vi "SetpointSetter.vi"() -> (1 "Arm Pos":T1, 3 "Shooter Servo Pos":T2)   [LabVIEW 2013]
uses:
  <vilib>/Utility/file.llb/Read From Spreadsheet File (DBL).vi
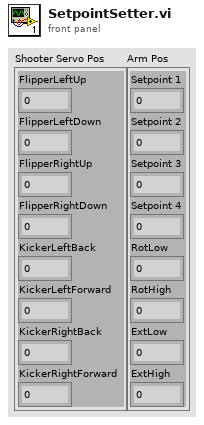
[diagram p1: front panel]
types:
  T1 = cluster{"Setpoint 1":dbl, "Setpoint 2":dbl, "Setpoint 3":dbl, "Setpoint 4":dbl, "RotLow":dbl, "RotHigh":dbl, "ExtLow":dbl, "ExtHigh":dbl}
  T2 = cluster{"FlipperLeftUp":dbl, "FlipperLeftDown":dbl, "FlipperRightUp":dbl, "FlipperRightDown":dbl, "KickerLeftBack":dbl, "KickerLeftForward":dbl, "KickerRightBack":dbl, "KickerRightForward":dbl}
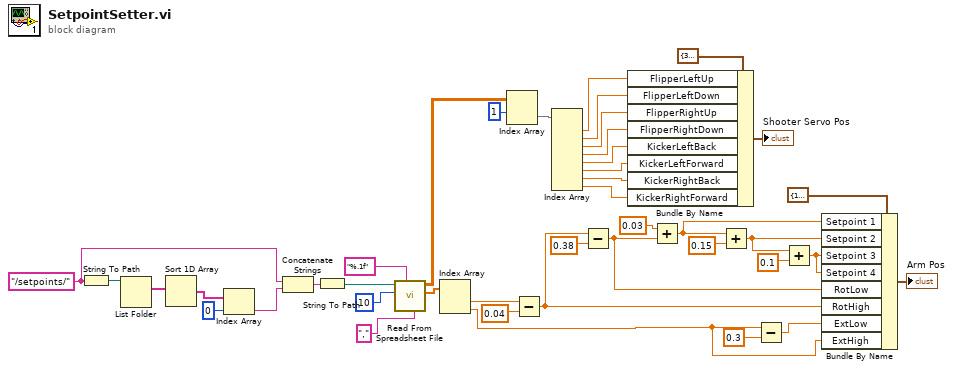
[diagram p0: block diagram]
diagram:
  w12 = "/setpoints/" ("string")
  n1 = String To Path(string=w12) -> (path=w10:path)
  n2 = List Folder(path=w10) -> (filenames=w9:string[])  [unwired: 1 in, 5 out]
  n3 = Sort 1D Array(array=w9) -> (sorted array=w8:string[])
  n4 = Index Array(array=w8, index=0) -> (element=w11:string)
  n5 = Concatenate Strings(w12, w11) -> (w6:string)
  n6 = String To Path(string=w6) -> (path=w7:path)
  n7 = call-poly <vilib>:"Read From Spreadsheet File.vi"("delimiter (\\t)"="," ("delimiter (\\t)"), "format (%.3f)"="%.1f", "number of rows (all:-1)"=10, "file path (dialog if empty)"=w7) -> ("first row"=w13:dbl[], "all rows"=w29:dbl[][])  [unwired: 1 in, 5 out]
  n8 = Index Array(array=w13) -> (element #1=w15:dbl, element #2=w28:dbl)  [unwired: 2 in]
  n9 = Index Array(array=w29, index (row)=1) -> (element=w32:dbl[])  [unwired: 1 in]
  n10 = Subtract(x=w15, y=0.04) -> (x-y=w17:dbl)
  n11 = Index Array(array=w32) -> (element #1=w33:dbl, element #2=w34:dbl, element #3=w35:dbl, element #4=w36:dbl, element #5=w37:dbl, element #6=w38:dbl, element #7=w39:dbl, element #8=w40:dbl)  [unwired: 8 in]
  n12 = Subtract(x=w17, y=0.38) -> (x-y=w19:dbl)
  n13 = Bundle By Name(cluster=T2 {"FlipperLeftUp"=30.0, "FlipperLeftDown"=115.0, "FlipperRightUp"=90.0, "FlipperRightDown"=90.0, "KickerLeftBack"=125.0, "KickerLeftForward"=70.0, "KickerRightBack"=45.0, "KickerRightForward"=100.0} ("ShooterServoPos"), "FlipperLeftUp"=w33, "FlipperLeftDown"=w34, "FlipperRightUp"=w35, "FlipperRightDown"=w36, "KickerLeftBack"=w37, "KickerLeftForward"=w38, "KickerRightBack"=w39, "KickerRightForward"=w40) -> (→"Shooter Servo Pos":T2)
  n14 = Add(x=0.03, y=w19) -> (x+y=w21:dbl)
  n15 = Add(x=w21, y=0.15) -> (x+y=w23:dbl)
  n16 = Subtract(x=w28, y=0.3) -> (x-y=w27:dbl)
  n17 = Add(x=w23, y=0.1) -> (x+y=w25:dbl)
  n18 = Bundle By Name(cluster=T1 {"Setpoint 1"=1.95, "Setpoint 2"=2.1, "Setpoint 3"=2.2, "Setpoint 4"=2.25, "RotLow"=1.92, "RotHigh"=2.3, "ExtLow"=1.87, "ExtHigh"=1.97} ("POTPositions"), "Setpoint 1"=w21, "Setpoint 2"=w23, "Setpoint 3"=w25, "Setpoint 4"=w25, "RotLow"=w19, "RotHigh"=w17, "ExtLow"=w27, "ExtHigh"=w28) -> (→"Arm Pos":T1)
